vi "getDeviceIP.vi"(11 "Device name":string) -> (3 "userID":string)   [LabVIEW 2020]
uses:
  Shared/MySQL/Preset Query Enum.ctl
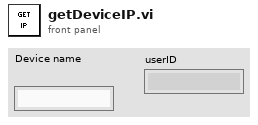
[diagram p1: front panel]
types:
  T1 = typedef "Preset Query Enum.ctl" = enum16{"Get Locations", "Get all IPs and MACs", "Get classes", "Get expt variables to set at scanstart for particular device", "Get expt devices and variables with start values", "Get expt devices and variables (with data to get)", "Get expt devices with data to get", "Get Expt devices and GUIs", "Get all devices basic properties", "Get Virtual Devices Core Info", "Get Expt names", "Get experiment basic properties", "Get experiment alarm variables", "Get MC Ports", "Get device network comm port", "Get devicetype lvclass path", "Get basic device properties", "Get Init Order", "Get all setable variables of a device", "Get device variable aliases", "Get force values of all settable variables", "Get all variables of a devicetype", "Get all variables of a device", "Get plotter details", "Get Saved Scans", "Get Scan Info", "GetGeneralGUIs", "Get expt for plotter", "Get plotter IDs from expt", "Get all devices", "Get all Virtual Devices", "Get all aliases", "Get variable and device info for Virtual Device", "GetItemLocatorIP", "Get IPs for GUIs", "Get DeviceType from Device", "GetLocalPortRange", "GetDevicePresetVariables", "Get Device Configuration", "GetAllPresetNames", "GetAllConfigurationNames", "GetPresetDeviceNames", "GetDeviceAliases", "GetDevicesOfClass"}
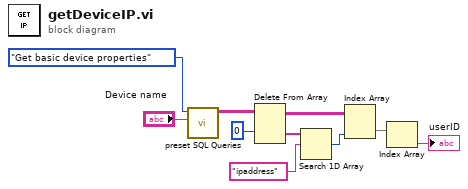
[diagram p0: block diagram]
diagram:
  n1 = call "preset SQL Queries.vi"("Device/Devicetype name\n/Plotter.id/ScanName#"="Device name", "Preset Query"=Preset_Query_Enum."Get basic device properties") -> ("data"=w4:string[][])  [unwired: 7 in, 2 out]
  n2 = Delete From Array(array=w4, index (row)=0) -> (deleted portion=w2:string[], array with subset deleted=w6:string[][])  [unwired: 2 in]
  n3 = Search 1D Array(1D array=w2, element="ipaddress") -> (index of element=w5:i32)  [unwired: 1 in]
  n4 = Index Array(array=w6, index (col)=w5) -> (element=w7:string[])  [unwired: 1 in]
  n5 = Index Array(array=w7) -> (element=→"userID":string)  [unwired: 1 in]
